vi "xiCam - StartAcquisition.vi"(8 "error in (no error)":errorcluster, 11 "xiCam In":refnum<k24>) -> (0 "error out":errorcluster, 3 "xiCam Out":refnum<k24>)   [LabVIEW 2018]
doc: "This function starts the data acquisition on the device.\n\n<b>void StartAcquisition()</b>"
uses:
  D:/codes labview/VisionLibrariesXimea/xiLib/xiLIB_64bit/xiLIB/xiCamLib/API/x64/xiApi.NETX64.dll
  API/x64/xiApi.NETX64.dll
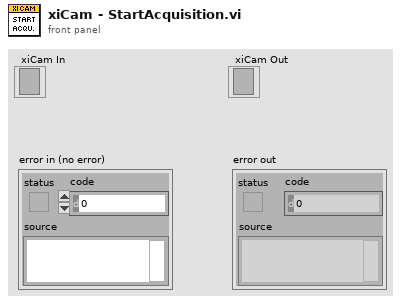
[diagram p1: front panel]
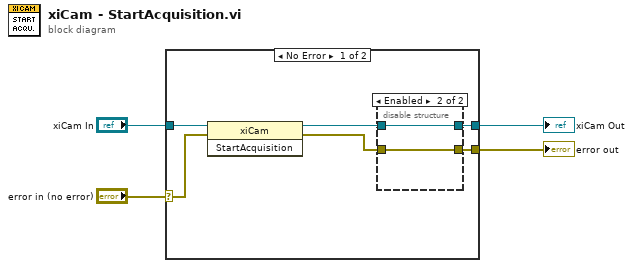
[diagram p0: block diagram]
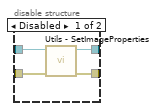
[diagram p2: hidden frame]
diagram:
  n1 = case shown="No Error" "error in (no error)" {
    selector: "error in (no error)" -> [w9 w17]
    tunnel: "xiCam In" -> [w10 w18]
    tunnel: [w6 w18] -> w2
    tunnel: [w5 w17] -> w1
    frame No Error {
      n2 = invoke class="xiCam" method="StartAcquisition"(reference=w10, error in=w9) -> (reference out=w8:refnum<k24>, error out=w7:errorcluster)  [unwired: 1 in, 1 out]
      n3 = disable-structure shown="Enabled" {
        disable-tunnel: w8 -> [w14 w16]
        disable-tunnel: w7 -> [w13 w15]
        disable-tunnel: [w12 w16] -> w6
        disable-tunnel: [w11 w15] -> w5
        frame Disabled {
          n4 = call "Utils - SetImageProperties.vi"("error in (no error)"=w13, "xiCam In"=w14) -> ("error out"=w11:errorcluster, "xiCam Out"=w12:refnum<k24>)  [unwired: 8 in]
        }
        frame Enabled {
        }
      }
    }
    frame Error {
    }
  }
  "error out" <- w1
  "xiCam Out" <- w2
